vi "Typedef.vi"() -> ()   [LabVIEW 2016, in "test_ValueSignal.lvlib"]
uses:
  test_ValueSignal.lvlib
  main/apis/Setup/GetVI/GetVIByPath.vi
  main/apis/Stimulus/ValueSignal/ValueSignalByPathString.vi
  main/apis/Assert/AssertControlValue/True.vi
  main/apis/Assert/AssertControlValue/Equal.vi
  <vilib>/addons/_JKI Toolkits/Caraya/classes/Test/Test.lvclass
  main/Drona.lvlib
  main/apis/Stimulus/ValueSignal/ValueSignal.lvlib
  main/apis/Assert/AssertControlValue/AssertControlValue.lvlib
  main/apis/Setup/GetVI/GetVI.lvlib
panel:
  out "error out":errorcluster
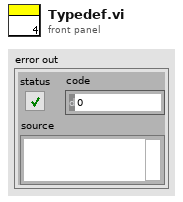
[diagram p1: front panel]
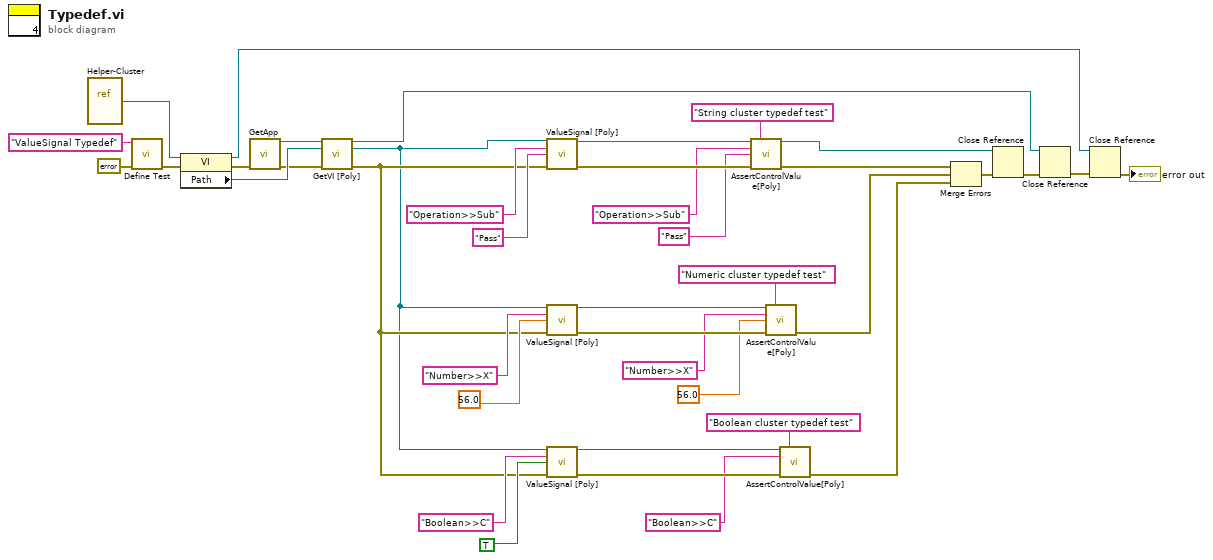
[diagram p0: block diagram]
diagram:
  n1 = vi-ref "Helper-Cluster.vi"() -> (w23:refnum<vi>)
  n2 = call <vilib>:"Define Test.vi"("error in (no error)"=errorcluster {"status"=FALSE, "code"=0, "source"=""}, "Label (VI Title)"="ValueSignal Typedef") -> ("error out"=w25:errorcluster)  [unwired: 9 in]
  n3 = property on="Property Node" class="VI"(reference=w23, error in=w25) -> (reference out=w19:refnum<vi>, error out=w29:errorcluster, "Path"=w28:path)
  n4 = call "GetApp.vi"("error in (no error)"=w29) -> ("Application Ref"=w30:refnum<vi>, "error out"=w27:errorcluster)  [unwired: 13 in]
  n5 = call-poly "GetVI [Poly].vi"("Application Ref in"=w30, "VI Path"=w28, "error in (no error)"=w27) -> ("Application Ref out"=w20:refnum<vi>, "VI Reference"=w21:refnum<vi>, "error out"=w22:errorcluster)  [unwired: 10 in]
  n6 = call-poly "ValueSignal [Poly].vi"("VI Reference In"=w21, "Control Name"="Operation>>Sub", "Value (Signaling)"="Pass" ("Control Name"), "error in"=w22) -> ("VI Reference Out"=w16:refnum<vi>, "error out"=w18:errorcluster)  [unwired: 10 in]
  n7 = call-poly "ValueSignal [Poly].vi"("VI Reference In"=w21, "Control Name"="Number>>X", "Value (Signaling)"=56.0, "error in"=w22) -> ("VI Reference Out"=w9:refnum<vi>, "error out"=w11:errorcluster)  [unwired: 10 in]
  n8 = call-poly "ValueSignal [Poly].vi"("VI Reference In"=w21, "Control Name"="Boolean>>C", "Value (Signaling)"=TRUE, "error in"=w22) -> ("VI Reference Out"=w2:refnum<vi>, "error out"=w5:errorcluster)  [unwired: 10 in]
  n9 = call-poly "AssertControlValue[Poly].vi"("VI Reference In"=w16, "Label"="String cluster typedef test" ("Label (VI Title)"), "Control Name"="Operation>>Sub", "Control Value"="Pass" ("Control Name"), "Error In"=w18) -> ("VI Reference Out"=w13:refnum<vi>, "Error Out"=w17:errorcluster)  [unwired: 9 in]
  n10 = call-poly "AssertControlValue[Poly].vi"("VI Reference In"=w9, "Label"="Numeric cluster typedef test" ("Label (VI Title)"), "Control Name"="Number>>X", "Control Value"=56.0, "Error In"=w11) -> ("Error Out"=w10:errorcluster)  [unwired: 9 in, 1 out]
  n11 = call-poly "AssertControlValue[Poly].vi"("VI Reference In"=w2, "Label"="Boolean cluster typedef test" ("Label (VI Title)"), "Control Name"="Boolean>>C", "Error In"=w5) -> ("Error Out"=w4:errorcluster)  [unwired: 10 in, 1 out]
  n12 = Merge Errors(w17, w10, w4) -> (w35:errorcluster)
  n13 = Close Reference(reference=w13, error in (no error)=w35) -> (error out=w38:errorcluster)
  n14 = Close Reference(reference=w20, error in (no error)=w38) -> (error out=w37:errorcluster)
  n15 = Close Reference(reference=w19, error in (no error)=w37) -> (error out=→"error out":errorcluster)
